vi "HW5p1_Task2_PPM_bartelmj (1).vi"() -> ()   [LabVIEW 2016]
panel:
  out "most severe category output":string
  out "diastolic category output":string
  out "stolic category output":string
  in  "diastolic(BPD)":dbl
  in  "systolic (BPS)":dbl
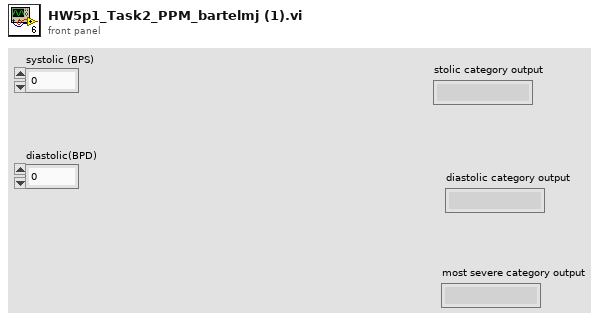
[diagram p1: front panel]
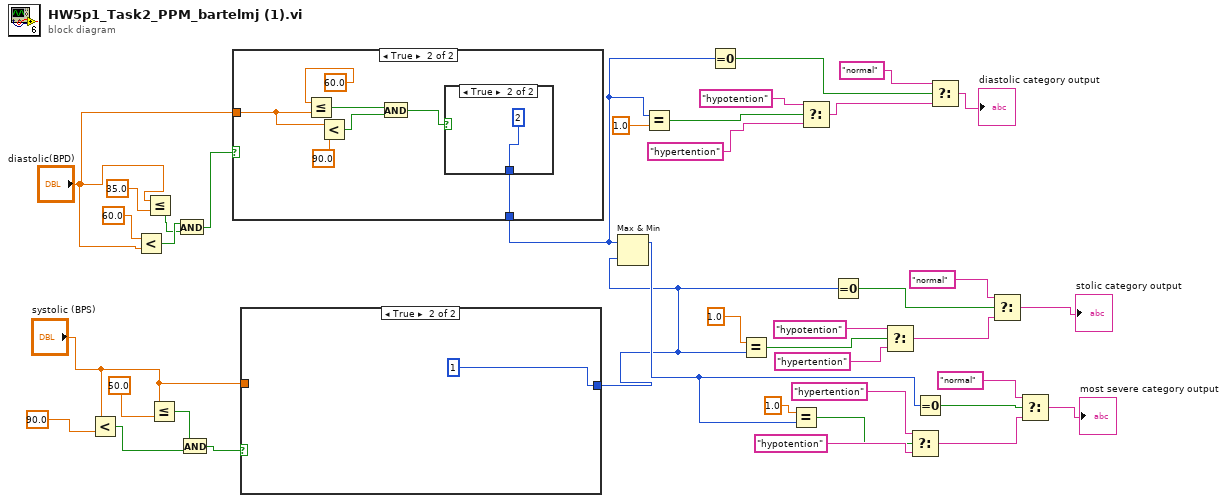
[diagram p0: block diagram]
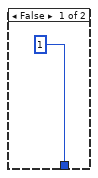
[diagram p2: hidden frame]
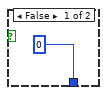
[diagram p3: hidden frame]
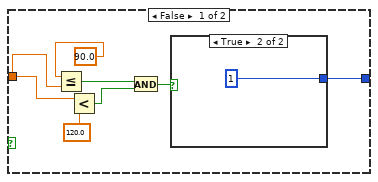
[diagram p4: hidden frame]
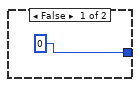
[diagram p5: hidden frame]
diagram:
  n1 = Less?(x="systolic (BPS)", y=90.0) -> (x < y?=w35:bool)
  n2 = Less?(x=60.0, y="diastolic(BPD)") -> (x < y?=w31:bool)
  n3 = Less Or Equal?(x="diastolic(BPD)", y=35.0) -> (x <= y?=w30:bool)
  n4 = Less Or Equal?(x="systolic (BPS)", y=50.0) -> (x <= y?=w36:bool)
  n5 = And(x=w31, y=w30) -> (x .and. y?=w29:bool)
  n6 = And(x=w36, y=w35) -> (x .and. y?=w34:bool)
  n7 = case shown="True" w29 {
    tunnel: "diastolic(BPD)" -> [_ w43]
    tunnel: [1 w41] -> w1
    frame False {
    }
    frame True {
      n8 = Less Or Equal?(x=60.0, y=w43) -> (x <= y?=w45:bool)
      n9 = Less?(x=w43, y=90.0) -> (x < y?=w44:bool)
      n10 = And(x=w45, y=w44) -> (x .and. y?=w42:bool)
      n11 = case shown="True" w42 {
        tunnel: [0 2] -> w41
        frame False {
        }
        frame True {
        }
      }
    }
  }
  n12 = case shown="True" w34 {
    tunnel: "systolic (BPS)" -> [w55 _]
    tunnel: [w50 1] -> w2
    frame False {
      n13 = Less Or Equal?(x=90.0, y=w55) -> (x <= y?=w53:bool)
      n14 = Less?(x=w55, y=120.0) -> (x < y?=w52:bool)
      n15 = And(x=w53, y=w52) -> (x .and. y?=w51:bool)
      n16 = case shown="True" w51 {
        tunnel: [0 1] -> w50
        frame False {
        }
        frame True {
        }
      }
    }
    frame True {
    }
  }
  n17 = Max & Min(x=w1, y=w2) -> (max(x,y)=w3:i32)  [unwired: 1 out]
  n18 = Equal?(x=w1, y=1.0) -> (x = y?=w22:bool)
  n19 = Equal To 0?(x=w1) -> (x = 0?=w25:bool)
  n20 = Equal?(x=1.0, y=w2) -> (x = y?=w13:bool)
  n21 = Equal?(x=1.0, y=w3) -> (x = y?=w5:bool)
  n22 = Select(t="hypotention", s=w22, f="hypertention") -> (s? t:f=w26:string)
  n23 = Equal To 0?(x=w2) -> (x = 0?=w16:bool)
  n24 = Select(t="hypotention", s=w13, f="hypertention") -> (s? t:f=w17:string)
  n25 = Select(t="hypertention", s=w5, f="hypotention") -> (s? t:f=w8:string)
  n26 = Equal To 0?(x=w3) -> (x = 0?=w9:bool)
  n27 = Select(t="normal", s=w25, f=w26) -> (s? t:f=→"diastolic category output":string)
  n28 = Select(t="normal", s=w16, f=w17) -> (s? t:f=→"stolic category output":string)
  n29 = Select(t="normal", s=w9, f=w8) -> (s? t:f=→"most severe category output":string)
